vi "Main.vi"() -> ()   [LabVIEW 2019]
uses:
  Controls/Calibration Plate Config.ctl
  Controls/Color.ctl
  <vilib>/vision/NI_Vision_Development_Module.lvlib
panel:
  out "Start(SGL)":bool
  out "Image":T1(plugin-control)
  in  "背景顏色":u32(colorbox)=16777215
  in  "圓點顏色":u32(colorbox)
  in  "圓點直間距 (cm)":dbl=2.0
  in  "圓點橫間距 (cm)":dbl=2.0
  in  "圓點直徑 (cm)":dbl=1.0
  in  "PPI":i32=300
  in  "寬度 (cm)":dbl=21.0
  in  "長度 (cm)":dbl=29.7
  # "圓心至圓心的間距"
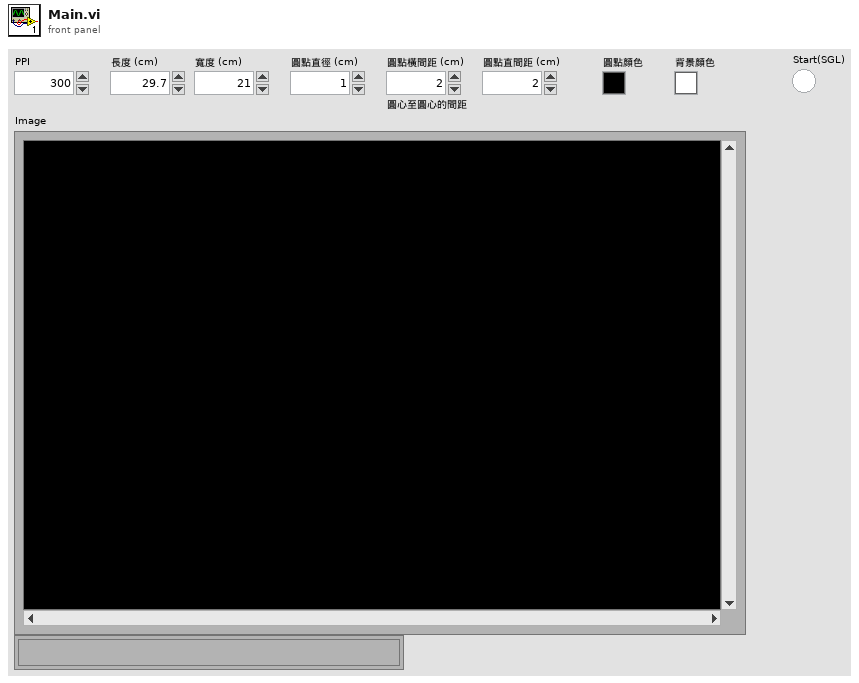
[diagram p1: front panel]
types:
  T1 = typedef "IMAQ Image.ctl" = refnum<image>
  T2 = typedef "Image Type" = u32
  T3 = typedef "Color.ctl" = cluster{"圓點顏色":u32, "背景顏色":u32}
  T4 = typedef "Calibration Plate Config.ctl" = cluster{"長度":dbl, "寬度":dbl, "圓點直徑":dbl, "圓點橫間距":dbl, "圓點直間距":dbl}
  T5 = cluster{"長度":i32, "寬度":i32, "圓點直徑":i32, "圓點橫間距":i32, "圓點直間距":i32}
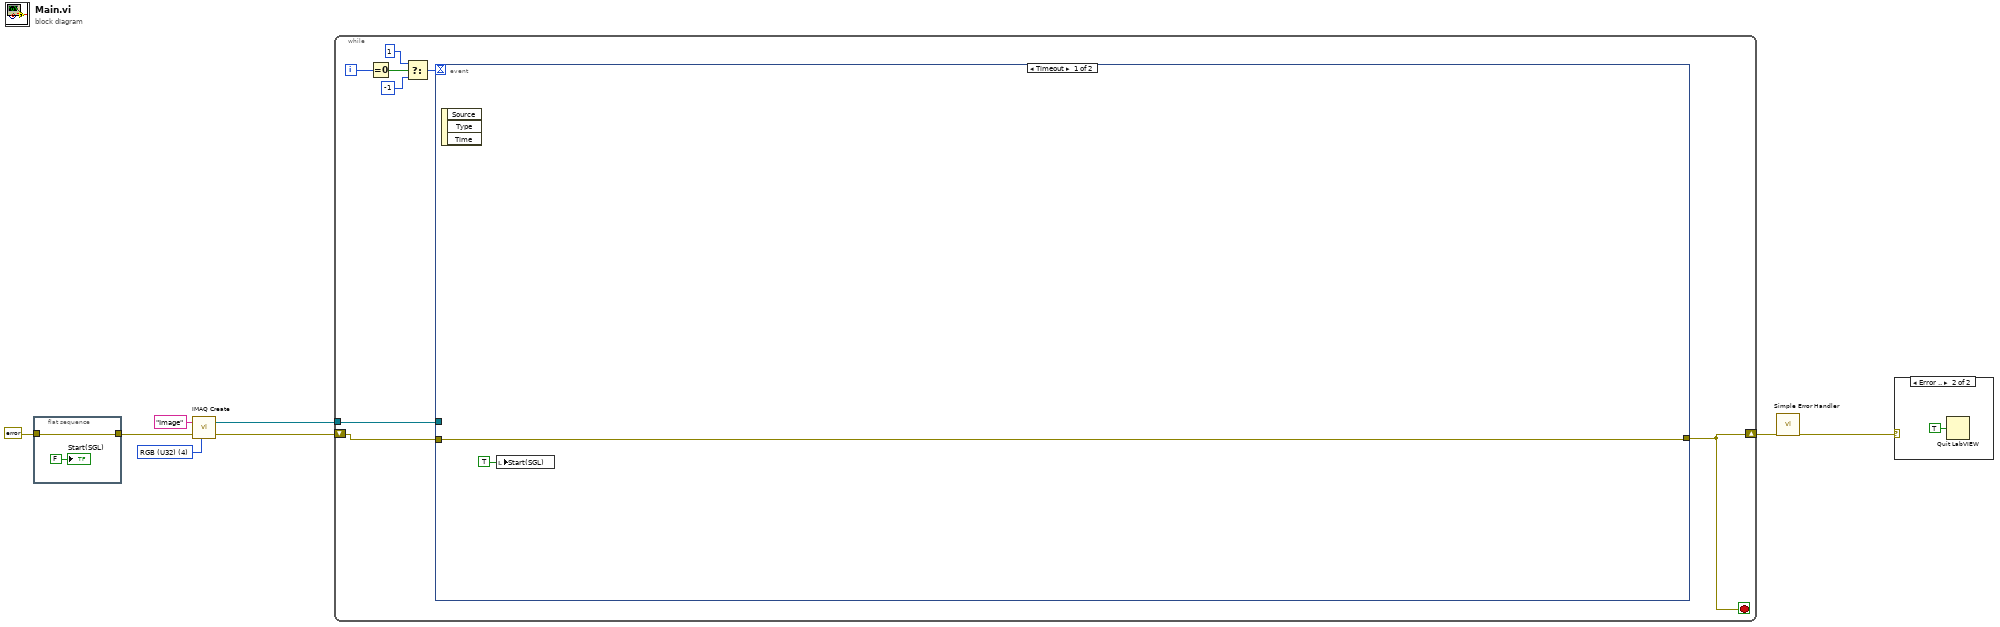
[diagram p0: block diagram]
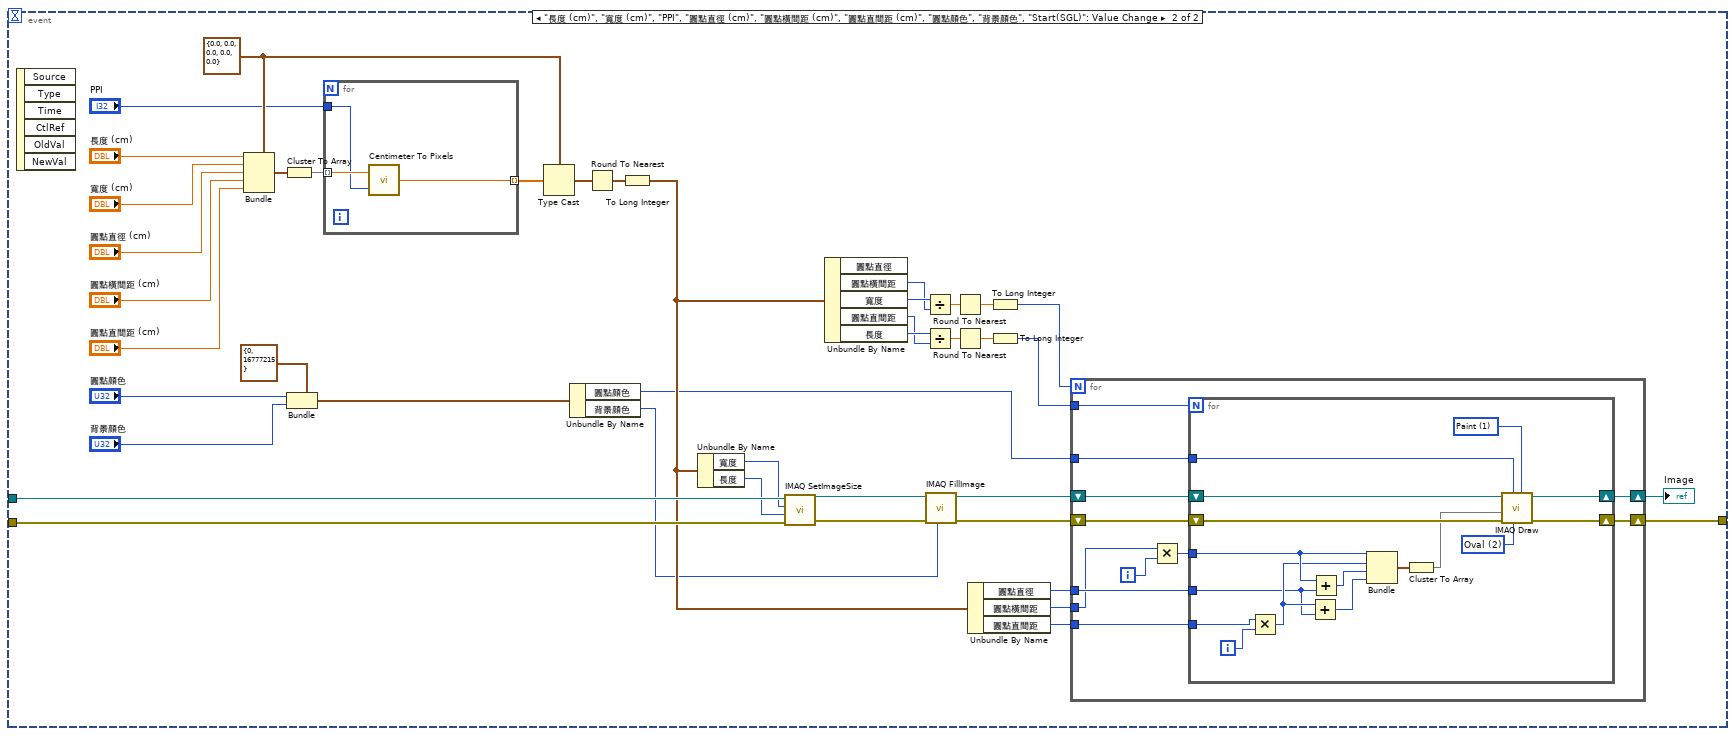
[diagram p2: hidden frame]
diagram:
  w5 = T2 4 items=["Grayscale (U8)", "Grayscale (I16)", "Grayscale (SGL)", "Complex (CSG)", "RGB (U32)", "HSL (U32)", "RGB (U64)", "Grayscale (U16)"] ("Image Type")
  n1 = flat-sequence {
    tunnel: [w9] -> w3
    tunnel: errorcluster {"status"=FALSE, "code"=0, "source"=""} ("error in (no error)") -> [w9]
    frame #0 {
      "Start(SGL)" <- FALSE ("Start(SGL)")
    }
  }
  n2 = call "IMAQ Create"("Image Name"="Image", "Image Type"=w5, "error in (no error)"=w3) -> ("New Image"=w4:T1, "error out"=w1:errorcluster)  [unwired: 2 in]
  n3 = while {
    shift-right: [w18] -> w7
    shift-left: w1 -> [w16]
    tunnel: w4 -> [w17]
    i -> [w15]
    stop <- w18 stop-if-true
    n4 = Equal To 0?(x=w15) -> (x = 0?=w14:bool)
    n5 = Select(t=1, s=w14, f=-1) -> (s? t:f=w11:i32)
    n6 = event shown="[0] Timeout" {
      selector: _ -> [_ _]
      dyn-events: _ -> [_ _]
      timeout: w11 -> [_ _]
      tunnel: [w20 w50] -> w18
      tunnel: w17 -> [_ w49]
      tunnel: w16 -> [w20 w48]
      event Timeout {
        n7 = event-data() -> ()  [unwired: 1 in, 3 out]
        n8 = local write "Start(SGL)"(TRUE ("Start(SGL)")) -> ()
      }
      event "長度 (cm)", "寬度 (cm)", "PPI", "圓點直徑 (cm)", "圓點橫間距 (cm)", "圓點直間距 (cm)", "圓點顏色", "背景顏色", "Start(SGL)": Value Change {
        w62 = T4 {"長度"=0.0, "寬度"=0.0, "圓點直徑"=0.0, "圓點橫間距"=0.0, "圓點直間距"=0.0}
        n9 = event-data() -> ()  [unwired: 1 in, 6 out]
        n10 = Bundle(cluster=w62, "長度"="長度 (cm)", "寬度"="寬度 (cm)", "圓點直徑"="圓點直徑 (cm)", "圓點橫間距"="圓點橫間距 (cm)", "圓點直間距"="圓點直間距 (cm)") -> (w56:T4)
        n11 = Cluster To Array(cluster=w56) -> (array=w55:dbl[])
        n12 = Bundle(cluster=T3 {"圓點顏色"=0, "背景顏色"=16777215} ("顏色"), "圓點顏色"="圓點顏色", "背景顏色"="背景顏色") -> (w43:T3)
        n13 = for {
          tunnel: w55 -> [w65] mode=indexing
          tunnel: "PPI" -> [w64]
          tunnel: [w63] -> w53 mode=indexing
          n14 = call "Centimeter To Pixels.vi"("PPI"=w64, "CM"=w65) -> ("Pixels"=w63:dbl)
        }
        n15 = Type Cast(type=w62, x=w53) -> (*(type *) &x=w52:T4)
        n16 = Unbundle By Name(w43) -> ("圓點顏色"=w24:u32, "背景顏色"=w23:u32)
        n17 = Round To Nearest(number=w52) -> (nearest integer value=w51:T4)
        n18 = To Long Integer(number=w51) -> (32bit integer=w47:T5)
        n19 = Unbundle By Name(w47) -> ("寬度"=w40:i32, "長度"=w39:i32)
        n20 = call "IMAQ SetImageSize"("error in (no error)"=w48, "Y Resolution"=w39, "X Resolution"=w40, "Image"=w49) -> ("error out"=w42:errorcluster, "Image Out"=w41:T1)  [unwired: 1 in]
        n21 = Unbundle By Name(w47) -> ("圓點橫間距"=w22:i32, "寬度"=w38:i32, "圓點直間距"=w21:i32, "長度"=w37:i32)  [unwired: 1 out]
        n22 = Divide(x=w38, y=w22) -> (x/y=w36:dbl)
        n23 = Divide(x=w37, y=w21) -> (x/y=w35:dbl)
        n24 = call "IMAQ FillImage"("Color Pixel Value"=w23, "error in (no error)"=w42, "Image"=w41) -> ("error out"=w31:errorcluster, "Image Out"=w30:T1)  [unwired: 7 in]
        n25 = Round To Nearest(number=w36) -> (nearest integer value=w34:dbl)
        n26 = Round To Nearest(number=w35) -> (nearest integer value=w33:dbl)
        n27 = Unbundle By Name(w47) -> ("圓點直徑"=w28:i32, "圓點橫間距"=w26:i32, "圓點直間距"=w27:i32)
        n28 = To Long Integer(number=w34) -> (32bit integer=w32:i32)
        n29 = To Long Integer(number=w33) -> (32bit integer=w29:i32)
        n30 = for {
          N: w32 -> [_]
          shift-right: [w73] -> w50
          shift-left: w31 -> [w76]
          shift-right: [w72] -> w25
          shift-left: w30 -> [w75]
          tunnel: w29 -> [w74]
          tunnel: w28 -> [w67]
          tunnel: w27 -> [w71]
          tunnel: w26 -> [w66]
          tunnel: w24 -> [w69]
          i -> [w68]
          n31 = Multiply(x=w66, y=w68) -> (x*y=w70:i32)
          n32 = for {
            N: w74 -> [_]
            shift-right: [w88] -> w73
            shift-left: w76 -> [w90]
            shift-right: [w87] -> w72
            shift-left: w75 -> [w89]
            tunnel: w67 -> [w83]
            tunnel: w71 -> [w77]
            tunnel: w70 -> [w86]
            tunnel: w69 -> [w79]
            i -> [w78]
            w91 = u16 1 items=["Frame", "Paint", "Invert Frame", "Invert Paint"] ("Draw Mode")
            w92 = u16 2 items=["Line", "Rectangle", "Oval"] ("Shape to draw")
            n33 = Multiply(x=w77, y=w78) -> (x*y=w84:i32)
            n34 = Add(x=w84, y=w83) -> (x+y=w82:i32)
            n35 = Add(x=w86, y=w83) -> (x+y=w85:i32)
            n36 = Bundle(w86, w84, w85, w82) -> (w81:cluster{i32, i32, i32, i32})  [unwired: 1 in]
            n37 = Cluster To Array(cluster=w81) -> (array=w80:i32[])
            n38 = call "IMAQ Draw"("Draw Mode"=w91, "Shape to draw"=w92, "Pixel Color"=w79, "error in (no error)"=w90, "Coordinates"=w80, "Image Src"=w89) -> ("error out"=w88:errorcluster, "Image Dst Out"=w87:T1)  [unwired: 4 in]
          }
        }
        "Image" <- w25
      }
    }
  }
  n39 = call <vilib>:"Simple Error Handler.vi"("error in (no error)"=w7) -> ("error out"=w8:errorcluster)  [unwired: 4 in, 4 out]
  n40 = case shown="Error .." w8 {
    frame No Error {
    }
    frame Error {
      n41 = Quit LabVIEW(quit? (T)=TRUE) -> ()
    }
  }
